vi "UTILITY 1D String Notifier.vi"(7 "Status":T1, 8 "error in (no error)":errorcluster, 10 "Set":string[](array[string]), 11 "name (unnamed)":string) -> (0 "error out":errorcluster, 3 "Array Output":string[](array[string]))   [LabVIEW 2014]
uses:
  Type Definitions/UTILITY Notifier.ctl
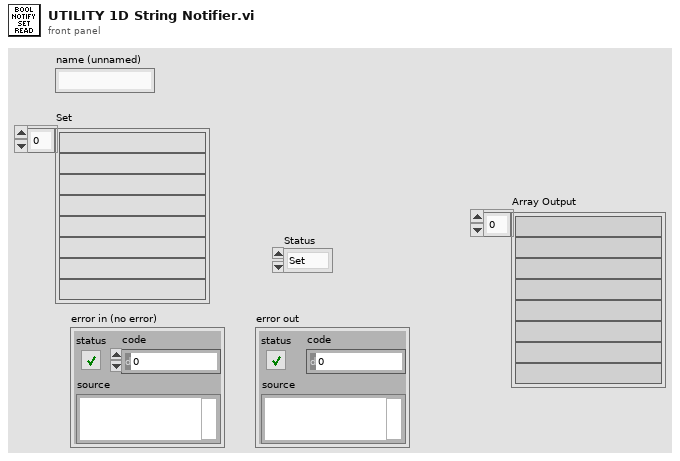
[diagram p1: front panel]
types:
  T1 = typedef "UTILITY Notifier.ctl" = enum16{"Set", "Read", "Release Ref"}
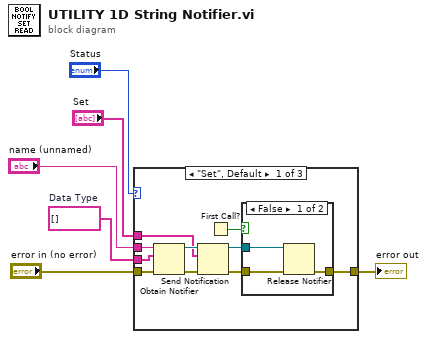
[diagram p0: block diagram]
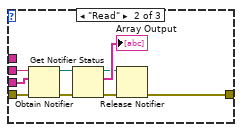
[diagram p3: hidden frame]
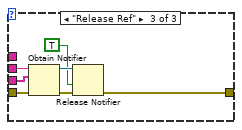
[diagram p4: hidden frame]
diagram:
  w2 = string[] []  # Data Type
  n1 = case shown="\"Set\", Default" "Status" {
    tunnel: [w9 w22 w31] -> w6
    tunnel: "error in (no error)" -> [w14 w27 w36]
    tunnel: "name (unnamed)" -> [w13 w26 w35]
    tunnel: w2 -> [w12 w25 w34]
    tunnel: "Set" -> [w11 _ _]
    frame "Set", Default {
      n2 = Obtain Notifier(name (unnamed)=w13, notification data type=w12, error in (no error)=w14) -> (notifier out=w15:refnum<notifier>, error out=w16:errorcluster)  [unwired: 1 in, 1 out]
      n3 = Send Notification(notification=w11, notifier=w15, error in (no error)=w16) -> (notifier out=w7:refnum<notifier>, error out=w10:errorcluster)
      n4 = First Call?() -> (First Call?: T/F=w8:bool)
      n5 = case shown="False" w8 {
        tunnel: w10 -> [w19 w20]
        tunnel: [w18 w20] -> w9
        tunnel: w7 -> [w17 _]
        frame False {
          n6 = Release Notifier(notifier=w17, error in (no error)=w19) -> (error out=w18:errorcluster)  [unwired: 1 in, 2 out]
        }
        frame True {
        }
      }
    }
    frame "Read" {
      n7 = Obtain Notifier(name (unnamed)=w26, notification data type=w25, error in (no error)=w27) -> (notifier out=w28:refnum<notifier>, error out=w29:errorcluster)  [unwired: 1 in, 1 out]
      n8 = Get Notifier Status(notifier=w28, error in (no error)=w29) -> (notifier out=w21:refnum<notifier>, current notification=→"Array Output":string[], error out=w23:errorcluster)  [unwired: 2 out]
      n9 = Release Notifier(notifier=w21, error in (no error)=w23) -> (error out=w22:errorcluster)  [unwired: 1 in, 2 out]
    }
    frame "Release Ref" {
      n10 = Obtain Notifier(name (unnamed)=w35, notification data type=w34, error in (no error)=w36) -> (notifier out=w33:refnum<notifier>, error out=w32:errorcluster)  [unwired: 1 in, 1 out]
      n11 = Release Notifier(notifier=w33, force destroy? (F)=TRUE, error in (no error)=w32) -> (error out=w31:errorcluster)  [unwired: 2 out]
    }
  }
  "error out" <- w6
